vi "_USB_CAN_BOARD_INFO_.vi"(11 "VCI_BOARD_INFO":T1) -> ()   [LabVIEW 2011]
doc: "ID=0x6005"
panel:
  in  "ok":bool
  out "str_hw_Type":string caption="硬件類型："
  out "str_Serial_Num":string caption="闆卡序列號："
  out "can_Num":u8 caption="can通道數："
  out "irq_Num":u16 caption="°åÝdÖÐ”à£º" format="0x%x"
  out "in_Ver":string caption="„Ó‘BŽì°æ±¾£º"
  out "dr_Ver":string caption="òŒ„Ó°æ±¾£º"
  out "fw_Ver":string caption="固件版本："
  out "hw_Ver":string caption="硬件版本："
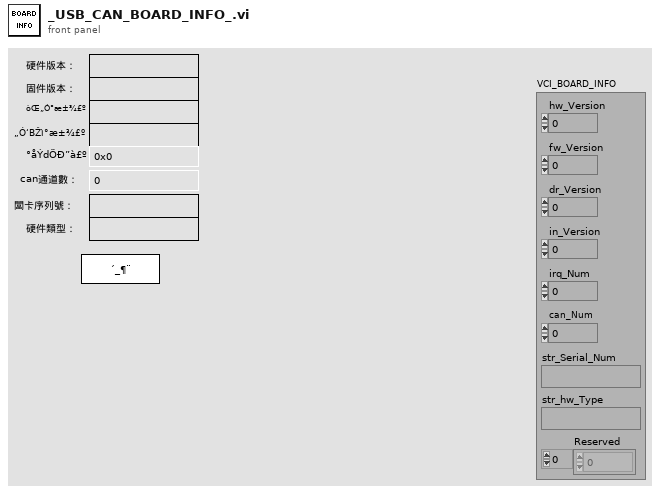
[diagram p1: front panel]
types:
  T1 = cluster{"hw_Version":u16, "fw_Version":u16, "dr_Version":u16, "in_Version":u16, "irq_Num":u16, "can_Num":u8, "str_Serial_Num":string, "str_hw_Type":string, "Reserved":u8[]}
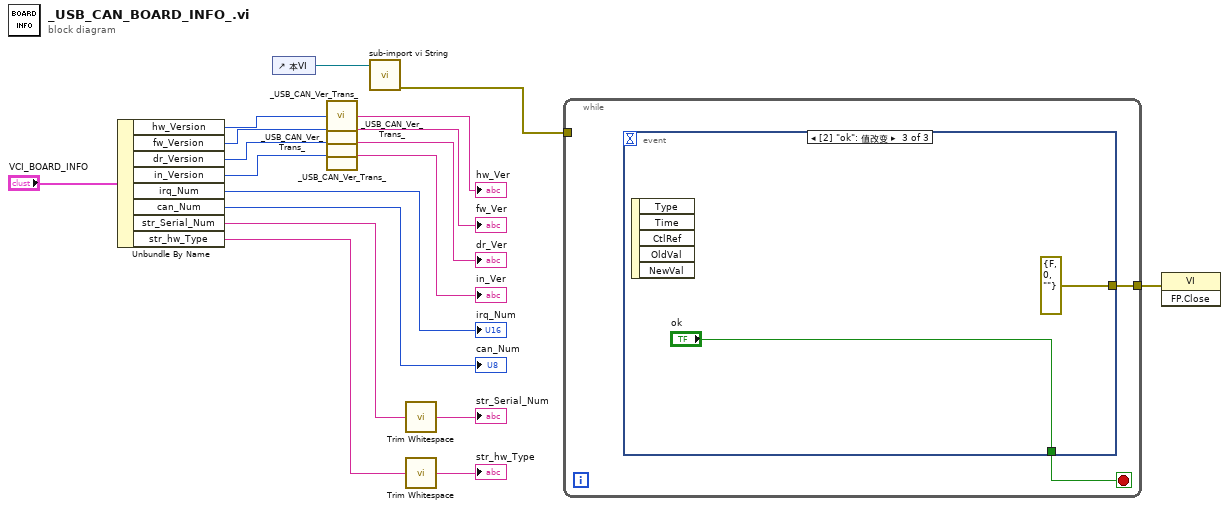
[diagram p0: block diagram]
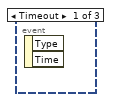
[diagram p2: hidden frame]
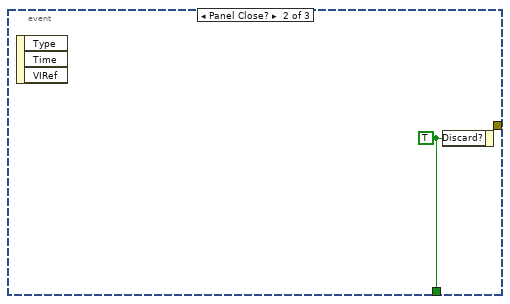
[diagram p3: hidden frame]
diagram:
  n1 = Unbundle By Name("VCI_BOARD_INFO") -> ("hw_Version"=w12:u16, "fw_Version"=w11:u16, "dr_Version"=w10:u16, "in_Version"=w9:u16, "irq_Num"=→"irq_Num":u16, "can_Num"=→"can_Num":u8, "str_Serial_Num"=w5:string, "str_hw_Type"=w3:string)
  n2 = control-ref of="本VI"() -> (w2:refnum<vi>)
  n3 = call "_USB_CAN_Ver_Trans_.vi"("u16Ver"=w12) -> ("strVer"=→"hw_Ver":string)
  n4 = call "_USB_CAN_Ver_Trans_.vi"("u16Ver"=w11) -> ("strVer"=→"fw_Ver":string)
  n5 = call "_USB_CAN_Ver_Trans_.vi"("u16Ver"=w10) -> ("strVer"=→"dr_Ver":string)
  n6 = call "_USB_CAN_Ver_Trans_.vi"("u16Ver"=w9) -> ("strVer"=→"in_Ver":string)
  n7 = call "sub-import vi String.vi"("vi ref"=w2) -> ("error out"=w1:errorcluster)  [unwired: 10 in]
  n8 = call <vilib>:"Trim Whitespace.vi"("string"=w5) -> ("trimmed string"=→"str_Serial_Num":string)  [unwired: 1 in]
  n9 = call <vilib>:"Trim Whitespace.vi"("string"=w3) -> ("trimmed string"=→"str_hw_Type":string)  [unwired: 1 in]
  n10 = while {
    tunnel: [w19] -> w18
    tunnel: w1 -> [_]
    stop <- w20 stop-if-true
    n11 = event shown="[2] \"ok\": 值改变" {
      selector: _ -> [_ _ _]
      dyn-events: _ -> [_ _ _]
      timeout: _ -> [_ _ _]
      tunnel: [_ w21 "ok"] -> w20
      tunnel: [_ _ errorcluster {"status"=FALSE, "code"=0, "source"=""} ("错误输入（无错误）")] -> w19
      event Timeout {
        n12 = event-data() -> ()  [unwired: 1 in, 2 out]
      }
      event Panel Close? {
        w21 = TRUE ("放弃？")
        n13 = event-data() -> ()  [unwired: 1 in, 3 out]
        n14 = event-data("Discard?"=w21) -> ()  [unwired: 1 in, 1 out]
      }
      event "ok": Value Change {
        n15 = event-data() -> ()  [unwired: 1 in, 5 out]
      }
    }
  }
  n16 = invoke class="VI" method="FP.Close"(error in=w18) -> ()  [unwired: 2 in, 3 out]
